vi "METIS_TestIOC_simple.vi"() -> ()   [LabVIEW 2020]
uses:
  2d31aa85-0ba4-4146-9dd6-b3e60546dde0.vi
  89720795-54a2-4534-9bbc-88a9e5af61a1.vi
  b2589dcb-5b22-4d43-a465-4351203ec25c.vi
  f4696480-f13b-456b-91c7-c20ebdb2ee9c.vi
  d910b247-ae28-4fff-85ad-f246d65b7ee6.vi
  <userlib>/caLab/Private/Put_I32-1D_PV-1D.vi
panel:
  in  "send":bool
  in  "stop":bool
  in  "Min":i32=10
  in  "Bin":i32=5
  in  "X":i32=10
  in  "Y":i32=10
  out "PV Errors":errorcluster[](array[cluster])=[{"status"=FALSE, "code"=7192, "source"="Virtual circuit disconnect"}]
  out "Status":bool=TRUE
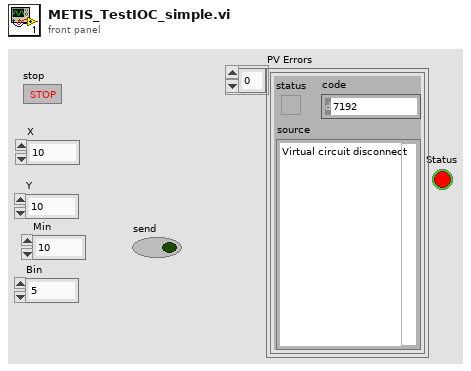
[diagram p1: front panel]
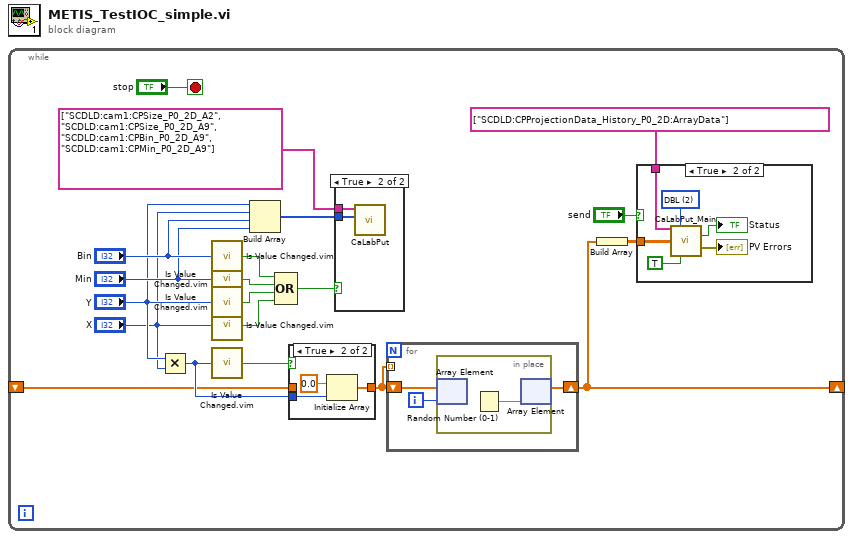
[diagram p0: block diagram]
diagram:
  n1 = while {
    shift-right: [w1] -> _
    shift-left: _ -> [w3]
    stop <- "stop" stop-if-true
    n2 = Multiply(x="Y", y="X") -> (x*y=w4:i32)
    n3 = call "Is Value Changed.vim"("value"="Bin") -> ("changed or first call?"=w12:bool)
    n4 = call "Is Value Changed.vim"("value"="Min") -> ("changed or first call?"=w11:bool)
    n5 = call "Is Value Changed.vim"("value"="Y") -> ("changed or first call?"=w16:bool)
    n6 = call "Is Value Changed.vim"("value"="X") -> ("changed or first call?"=w15:bool)
    n7 = call "Is Value Changed.vim"("value"=w4) -> ("changed or first call?"=w5:bool)
    n8 = Build Array("Y", "X", "Bin", "Min") -> (w9:i32[])
    n9 = Compound Arithmetic op=OR(w12, w11, w16, w15) -> (w10:bool)
    n10 = case shown="True" w5 {
      tunnel: w4 -> [_ w27]
      tunnel: [w25 w26] -> w2
      tunnel: w3 -> [w25 _]
      frame False {
      }
      frame True {
        n11 = Initialize Array(0.0 ("element"), w27) -> (w26:dbl[])
      }
    }
    n12 = case shown="True" w10 {
      tunnel: w9 -> [_ w30]
      tunnel: string[] ["SCDLD:cam1:CPSize_P0_2D_A2", "SCDLD:cam1:CPSize_P0_2D_A9", "SCDLD:cam1:CPBin_P0_2D_A9", "SCDLD:cam1:CPMin_P0_2D_A9"] -> [_ w29]
      frame False {
      }
      frame True {
        n13 = call-poly <userlib>:"CaLabPut.vi"("Values"=w30, "PV Names"=w29) -> ()  [unwired: 6 in, 4 out]
      }
    }
    n14 = for {
      shift-right: [w21] -> w1
      shift-left: w2 -> [w23]
      tunnel: w2 -> [_] mode=indexing
      i -> [w22]
      n15 = in-place {
        n16 = in-place-array #1(w23, w22) -> ()  [unwired: 1 out]
        n17 = Random Number (0-1)() -> (number: 0 to 1=w24:dbl)
        n18 = in-place-array #1(w24) -> (w21:dbl[])  [unwired: 1 out]
      }
    }
    n19 = Build Array(w1) -> (w20:dbl[][])
    n20 = case shown="True" "send" {
      tunnel: w20 -> [_ w36]
      tunnel: string[] ["SCDLD:CPProjectionData_History_P0_2D:ArrayData"] -> [_ w33]
      frame False {
      }
      frame True {
        w32 = 2 items=["String", "SGL", "DBL", "I8", "I16", "I32", "I64"] ("Data Type")
        n21 = call <userlib>:"CaLabPut_Main.vi"("PV Names"=w33, "Data Type"=w32, "Values [DBL]"=w36, "Synchronous"=TRUE) -> ("Status"=→"Status":bool, "PV Errors"=→"PV Errors":errorcluster[])  [unwired: 8 in, 2 out]
      }
    }
  }
